vi "[3조_오전반]LabVIEW angry ver..vi"() -> ()   [LabVIEW 2019]
uses:
  <vilib>/DAQmx/read.llb/DAQmx Read (Analog Wfm 1Chan NSamp).vi
  <vilib>/DAQmx/create/channels.llb/DAQmx Create Channel (AI-Voltage-Basic).vi
  <vilib>/DAQmx/configure/timing.llb/DAQmx Timing (Sample Clock).vi
  <vilib>/DAQmx/miscellaneous.llb/DAQmx Fill In Error Info.vi
  <vilib>/measure/matone.llb/Extract Single Tone Information 1 Chan.vi
  <vilib>/measure/NI_MABase.lvlib
  <vilib>/measure/NI_MAPro.lvlib
panel:
  in  "정지 2":bool
  in  "?":tag
  in  "?":enum16{"충격", "소리"}(ring)
  out "Vp-p (V)":dbl
  out "Vp-p (V)":dbl
  out "주파수 (Hz)":dbl
  out "주기 (ms)":dbl
  out "진폭 (V)":dbl
  out "주파수 (Hz)":dbl
  out "주기 (ms)":dbl
  out "DC Offset(V)":dbl
  out "진폭 (V)":dbl
  in  "?":enum16{"GND", "DC", "AC"}(ring)
  in  "?":bool
  in  "?":tag
  out "?":waveform(dbl)(graph)
  # "애정이의\nOscilloscope"
  # "--- Cursor ---"
  # "- Measure -"
  # "DC Mode"
  # "AC Mode"
  # "커서 방향키"
  # "좌/우 버튼: 좌/우 방향으로 커서 움직임\n0.002씩 움직이며 그에 해당하는 Y값 보여줌"
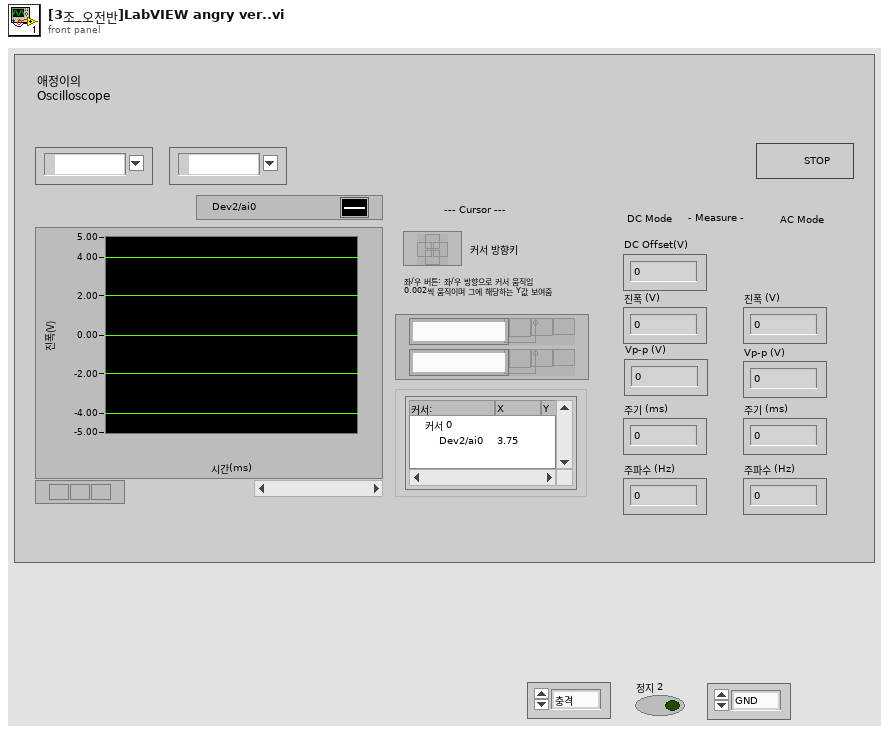
[diagram p1: front panel]
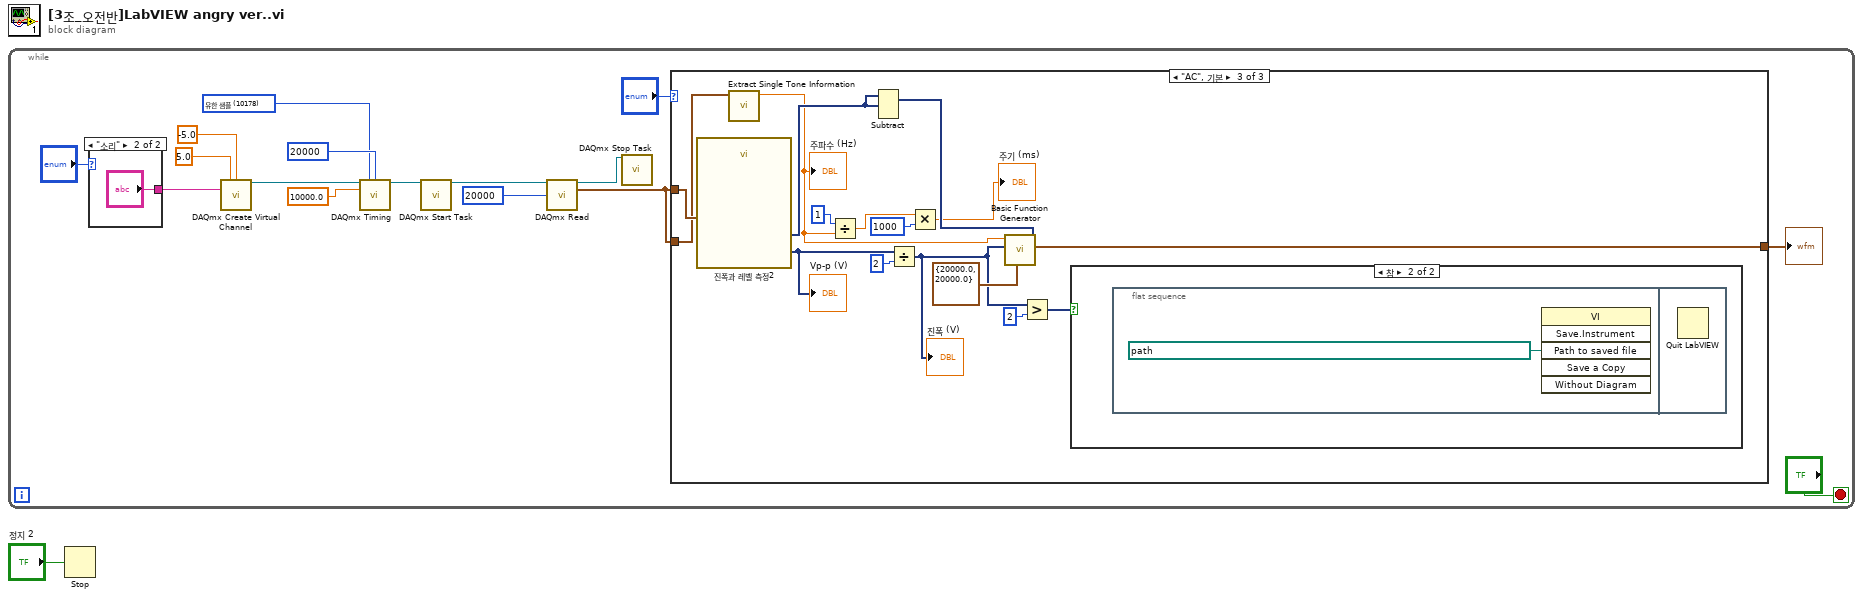
[diagram p0: block diagram]
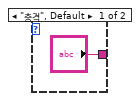
[diagram p2: hidden frame]
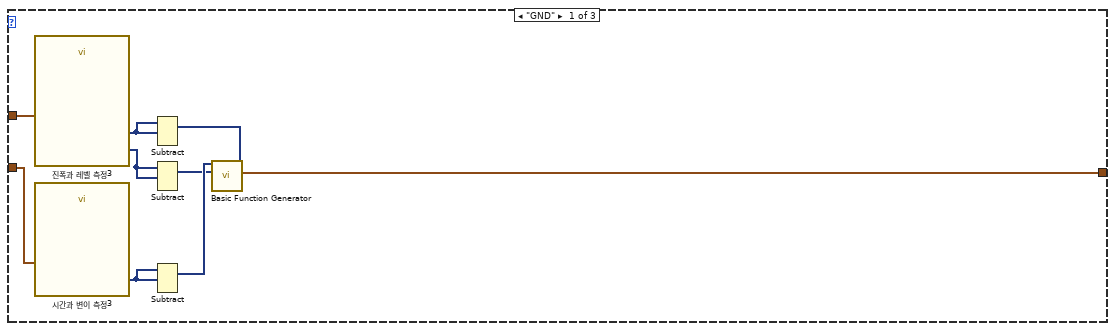
[diagram p3: hidden frame]
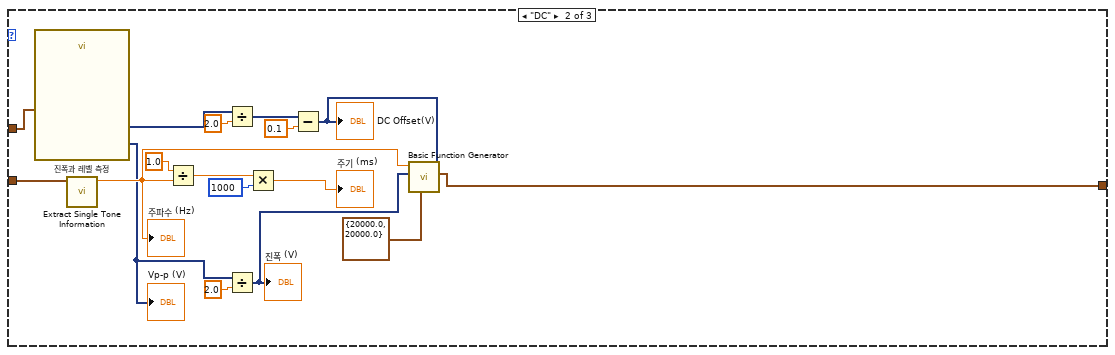
[diagram p4: hidden frame]
diagram:
  n1 = while {
    stop <- "?" stop-if-true
    w9 = 10178 items=["유한 샘플"=10178, "연속 샘플"=10123, "하드웨어 타이밍에 의한 단일 포인트"=12522] ("sample mode")
    n2 = case shown="\"소리\"" "?" {
      tunnel: ["?" "?"] -> w2
      frame "충격", Default {
      }
      frame "소리" {
      }
    }
    n3 = call-poly <vilib>:"DAQmx Create Virtual Channel.vi"("maximum value"=5.0, "minimum value"=-5.0, "physical channels"=w2) -> ("task out"=w17:refnum<k21>)  [unwired: 11 in, 1 out]
    n4 = call-poly <vilib>:"DAQmx Timing.vi"("task/channels in"=w17, "sample mode"=w9, "samples per channel"=20000, "rate"=10000.0) -> ("task out"=w16:refnum<k21>)  [unwired: 10 in, 1 out]
    n5 = call <vilib>:"DAQmx Start Task.vi"("task/channels in"=w16) -> ("task out"=w15:refnum<k21>)  [unwired: 13 in, 1 out]
    n6 = call-poly <vilib>:"DAQmx Read.vi"("task/channels in"=w15, "number of samples per channel"=20000) -> ("task out"=w14:refnum<k21>, "data"=w6:waveform(dbl))  [unwired: 11 in, 1 out]
    n7 = call <vilib>:"DAQmx Stop Task.vi"("task/channels in"=w14) -> ()  [unwired: 13 in, 2 out]
    n8 = case shown="\"AC\", 기본" "?" {
      tunnel: w6 -> [w27 w40 w54]
      tunnel: w6 -> [w22 w41 w57]
      tunnel: [w28 w45 w61] -> w5
      frame "GND" {
        n9 = call "진폭과 레벨 측정3"("Signals"=w22) -> ("Mean (DC)"=w21:dynamicdata, "Peak to Peak"=w20:dynamicdata)  [unwired: 12 in, 1 out]
        n10 = call "시간과 변이 측정3"("Signals"=w27) -> ("Frequency"=w26:dynamicdata)  [unwired: 9 in, 1 out]
        n11 = Subtract(1:w21, 2:w21) -> (0:w23:dynamicdata)  [unwired: 1 in, 1 out]
        n12 = Subtract(1:w20, 2:w20) -> (0:w24:dynamicdata)  [unwired: 1 in, 1 out]
        n13 = Subtract(1:w26, 2:w26) -> (0:w25:dynamicdata)  [unwired: 1 in, 1 out]
        n14 = call <vilib>:"Basic Function Generator.vi"("offset"=w23, "amplitude"=w24, "frequency"=w25) -> ("signal out"=w28:waveform(dbl))  [unwired: 6 in, 2 out]
      }
      frame "DC" {
        n15 = call "진폭과 레벨 측정"("Signals"=w41) -> ("Mean (DC)"=w32:dynamicdata, "Peak to Peak"=w34:dynamicdata)  [unwired: 12 in, 1 out]
        "Vp-p (V)" <- w34
        n16 = call-poly <vilib>:"Extract Single Tone Information.vi"("time signal in"=w40) -> ("detected frequency"=w39:dbl)  [unwired: 5 in, 5 out]
        "주파수 (Hz)" <- w39
        n17 = Divide(x=1.0, y=w39) -> (x/y=w37:dbl)
        n18 = Divide(x=w32, y=2.0) -> (x/y=w30:dynamicdata)
        n19 = Divide(x=w34, y=2.0) -> (x/y=w42:dynamicdata)
        "진폭 (V)" <- w42
        n20 = Multiply(x=w37, y=1000) -> (x*y=→"주기 (ms)":dbl)
        n21 = Subtract(x=w30, y=0.1) -> (x-y=w29:dynamicdata)
        "DC Offset(V)" <- w29
        n22 = call <vilib>:"Basic Function Generator.vi"("offset"=w29, "sampling info"=cluster{"Fs":dbl, "#s":dbl} {"Fs"=20000.0, "#s"=20000.0}, "amplitude"=w42, "frequency"=w39) -> ("signal out"=w45:waveform(dbl))  [unwired: 5 in, 2 out]
      }
      frame "AC", Default {
        n23 = call "진폭과 레벨 측정2"("Signals"=w57) -> ("Mean (DC)"=w56:dynamicdata, "Peak to Peak"=w50:dynamicdata)  [unwired: 12 in, 1 out]
        "Vp-p (V)" <- w50
        n24 = call-poly <vilib>:"Extract Single Tone Information.vi"("time signal in"=w54) -> ("detected frequency"=w49:dbl)  [unwired: 5 in, 5 out]
        "주파수 (Hz)" <- w49
        n25 = Divide(x=1, y=w49) -> (x/y=w52:dbl)
        n26 = Subtract(1:w56, 2:w56) -> (0:w60:dynamicdata)  [unwired: 1 in, 1 out]
        n27 = Divide(x=w50, y=2) -> (x/y=w48:dynamicdata)
        "진폭 (V)" <- w48
        n28 = Multiply(x=w52, y=1000) -> (x*y=→"주기 (ms)":dbl)
        n29 = call <vilib>:"Basic Function Generator.vi"("offset"=w60, "sampling info"=cluster{"Fs":dbl, "#s":dbl} {"Fs"=20000.0, "#s"=20000.0}, "amplitude"=w48, "frequency"=w49) -> ("signal out"=w61:waveform(dbl))  [unwired: 5 in, 2 out]
        n30 = Greater?(x=w48, y=2) -> (0:w46:dynamicdata)
        n31 = case shown="참" w46 {
          frame False {
          }
          frame True {
            n32 = flat-sequence {
              frame #0 {
                n33 = invoke class="VI" method="Save.Instrument"("Path to saved file"=path "C:/Users/구윤정/Desktop/기초전자공학/[3조_오전반]오실로스코프.vi" ("저장된 파일 경로")) -> ()  [unwired: 5 in, 6 out]
              }
              frame #1 {
                n34 = Quit LabVIEW() -> ()  [unwired: 1 in]
              }
            }
          }
        }
      }
    }
    "?" <- w5
  }
  n35 = Stop(stop? (T)="정지 2") -> ()
